vi "jump abs.vi"(8 "error in (no error)":errorcluster, 10 "y":i16, 11 "x":i16) -> (0 "error out":errorcluster)   [LabVIEW 2015, in "SCANalone4x64.lvlib"]
doc: "__declspec(dllimport) void __stdcall jump_abs(short x, short y);"
uses:
  <userlib>/SCANalone4x64/SCANalone4x64.lvlib
  <userlib>/SCANalone4x64/SCANalone4x64.dll
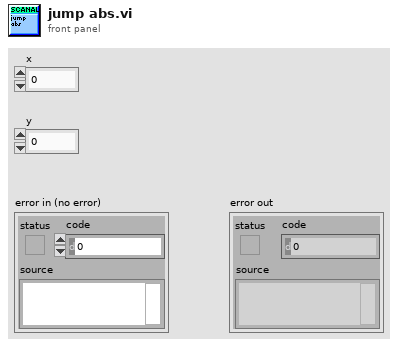
[diagram p1: front panel]
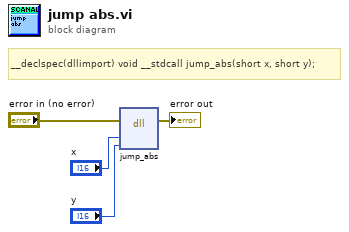
[diagram p0: block diagram]
diagram:
  # "__declspec(dllimport) void __stdcall jump_abs(short x, short y);"
  n1 = dll-call lib="C:/Program Files/National Instruments/LabVIEW 2015/user.lib/SCANalone4x64/SCANalone4x64.*" fn="jump_abs"(error in="error in (no error)", "x"="x", "y"="y") -> (error out=→"error out":errorcluster)  [unwired: 5 in, 1 out]
